vi "Extract Court (SubVI).vi"(2 "error in (no error)":errorcluster, 3 "AVI Path":path) -> (0 "error out":errorcluster, 1 "Court pixels out":u8[][](array[numeric]))   [LabVIEW 2014]
uses:
  <vilib>/vision/NI_Vision_Development_Module.lvlib
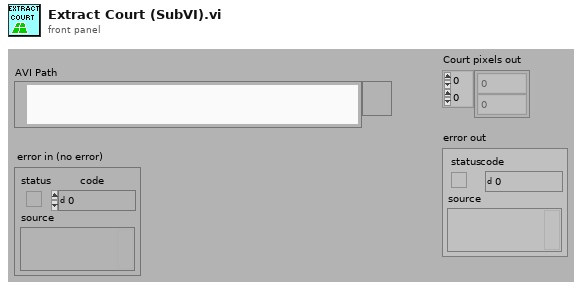
[diagram p1: front panel]
types:
  T1 = enum32{"AutoM", "Close", "Dilate", "Erode", "Gradient", "Gradient in", "Gradient out", "HitMiss", "Open", "PClose", "POpen", "Thick", "Thin"}
  T2 = typedef "Image Type" = u32
  T3 = typedef "AviRefnum.ctl" = refnum<k1>
  T4 = typedef "IMAQ Image.ctl" = refnum<image>
  T5 = cluster{"Starting Value":sgl, "Incremental Value":sgl, "Histogram":u32[]}
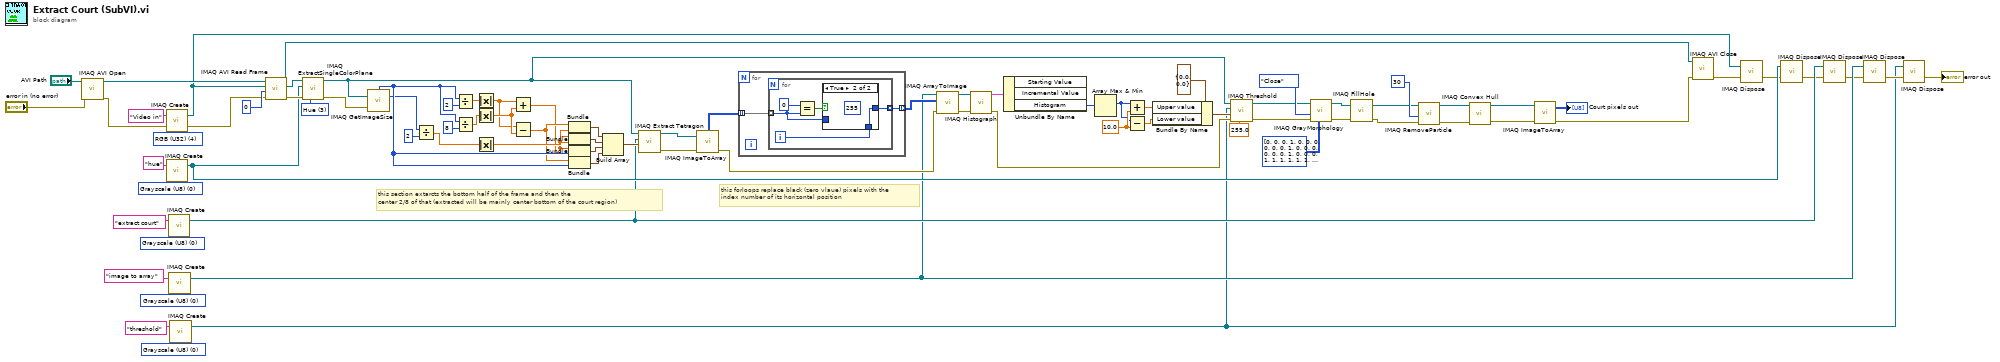
[diagram p0: block diagram]
diagram:
  w37 = 3 items=["Red", "Green", "Blue", "Hue", "Saturation", "Luminance", "Value", "Intensity"] ("Color Plane")
  w63 = sgl 10.0 ("Upper value")
  w31 = T2 0 items=["Grayscale (U8)", "Grayscale (I16)", "Grayscale (SGL)", "Complex (CSG)", "RGB (U32)", "HSL (U32)", "RGB (U64)", "Grayscale (U16)"] ("Image Type")
  w33 = T2 0 items=["Grayscale (U8)", "Grayscale (I16)", "Grayscale (SGL)", "Complex (CSG)", "RGB (U32)", "HSL (U32)", "RGB (U64)", "Grayscale (U16)"] ("Image Type")
  w29 = T2 0 items=["Grayscale (U8)", "Grayscale (I16)", "Grayscale (SGL)", "Complex (CSG)", "RGB (U32)", "HSL (U32)", "RGB (U64)", "Grayscale (U16)"] ("Image Type")
  w28 = T2 0 items=["Grayscale (U8)", "Grayscale (I16)", "Grayscale (SGL)", "Complex (CSG)", "RGB (U32)", "HSL (U32)", "RGB (U64)", "Grayscale (U16)"] ("Image Type")
  w26 = T2 4 items=["Grayscale (U8)", "Grayscale (I16)", "Grayscale (SGL)", "Complex (CSG)", "RGB (U32)", "HSL (U32)", "RGB (U64)", "Grayscale (U16)"] ("Image Type")
  # "this forloops replace black (zero vlaue) pixels with the \nindex number of its horizontal position"
  # "this section extarcts the bottom half of the frame and then the \ncenter 2/8 of that (extracted will be mainly center bottom of the court region)"
  n1 = call "IMAQ AVI Open"("error in (no error)"="error in (no error)", "AVI Path"="AVI Path") -> ("error out"=w36:errorcluster, "Avi Refnum"=w35:T3)  [unwired: 8 in]
  n2 = call "IMAQ Create"("Image Name"="Video in", "Image Type"=w26, "error in (no error)"=w36) -> ("New Image"=w21:T4, "error out"=w25:errorcluster)  [unwired: 2 in]
  n3 = call "IMAQ Create"("Image Name"="hue", "Image Type"=w28) -> ("New Image"=w20:T4)  [unwired: 3 in, 1 out]
  n4 = call "IMAQ Create"("Image Name"="extract court", "Image Type"=w33) -> ("New Image"=w19:T4)  [unwired: 3 in, 1 out]
  n5 = call "IMAQ Create"("Image Name"="image to array", "Image Type"=w31) -> ("New Image"=w18:T4)  [unwired: 3 in, 1 out]
  n6 = call "IMAQ Create"("Image Name"="threshold", "Image Type"=w29) -> ("New Image"=w2:T4)  [unwired: 3 in, 1 out]
  n7 = call "IMAQ AVI Read Frame"("error in (no error)"=w25, "Frame Number"=u32 0, "Image"=w21, "Avi Refnum"=w35) -> ("error out"=w68:errorcluster, "Image Out"=w77:T4, "Avi Refnum (duplicate)"=w22:T3)  [unwired: 4 in, 1 out]
  n8 = call "IMAQ ExtractSingleColorPlane"("Color Plane"=w37, "error in (no error)"=w68, "Image Dst"=w20, "Image Src"=w77) -> ("error out"=w69:errorcluster, "Image Dst Out"=w5:T4)  [unwired: 6 in]
  n9 = call "IMAQ GetImageSize"("Image"=w5, "error in (no error)"=w69) -> ("Y Resolution"=w39:i32, "X Resolution"=w55:i32)  [unwired: 2 in, 1 out]
  n10 = Divide(x=w39, y=2) -> (x/y=w44:dbl)
  n11 = Divide(x=w55, y=2) -> (x/y=w47:dbl)
  n12 = Divide(x=w55, y=8) -> (x/y=w46:dbl)
  n13 = Absolute Value(x=w47) -> (abs(x)=w48:dbl)
  n14 = Absolute Value(x=w46) -> (abs(x)=w49:dbl)
  n15 = Absolute Value(x=w44) -> (abs(x)=w45:dbl)
  n16 = Add(x=w48, y=w49) -> (x+y=w42:dbl)
  n17 = Subtract(x=w48, y=w49) -> (x-y=w43:dbl)
  n18 = Bundle(w43, w45) -> (w50:cluster{dbl, dbl})  [unwired: 1 in]
  n19 = Bundle(w42, w45) -> (w51:cluster{dbl, dbl})  [unwired: 1 in]
  n20 = Bundle(w42, "X Resolution"=w55) -> (w52:cluster{dbl, "X Resolution":i32})  [unwired: 1 in]
  n21 = Bundle(w43, "X Resolution"=w55) -> (w53:cluster{dbl, "X Resolution":i32})  [unwired: 1 in]
  n22 = Build Array(w50, w51, w52, w53) -> (w54:cluster{dbl, "X Resolution":dbl}[])
  n23 = call-poly "IMAQ Extract Tetragon"("Tetragon"=w54, "Image Dst"=w19, "Image Src"=w5) -> ("error out"=w65:errorcluster, "Image Dst Out"=w6:T4)  [unwired: 7 in]
  n24 = call "IMAQ ImageToArray"("error in (no error)"=w65, "Image"=w6) -> ("error out"=w83:errorcluster, "Image Pixels (U8)"=w56:u8[][])  [unwired: 2 in, 3 out]
  n25 = for {
    tunnel: w56 -> [w85] mode=indexing
    tunnel: [w84] -> w57 mode=indexing
    n26 = for {
      tunnel: w85 -> [w87] mode=indexing
      tunnel: [w88] -> w84 mode=indexing
      i -> [w86]
      n27 = Equal?(x=u8 0, y=w87) -> (x = y?=w89:bool)
      n28 = case shown="True" w89 {
        tunnel: [w91 w92] -> w88
        tunnel: w87 -> [w91 _]
        tunnel: w86 -> [_ w92]
        frame False {
        }
        frame True {
          (unwired) u8 255 ("x")
        }
      }
    }
  }
  n29 = call "IMAQ ArrayToImage"("error in (no error)"=w83, "Image Pixels (U8)"=w57, "Image"=w18) -> ("error out"=w70:errorcluster, "Image Out"=w4:T4)  [unwired: 7 in]
  n30 = call "IMAQ Histograph"("error in (no error)"=w70, "Image"=w4) -> ("error out"=w71:errorcluster, "Histogram Graph"=w58:T5)  [unwired: 6 in, 2 out]
  n31 = Unbundle By Name(w58) -> ("Histogram"=w59:u32[])  [unwired: 2 out]
  n32 = Array Max & Min(array=w59) -> (max index (indices)=w60:i32)  [unwired: 3 out]
  n33 = Add(x=w60, y=w63) -> (x+y=w66:sgl)
  n34 = Subtract(x=w60, y=w63) -> (x-y=w67:sgl)
  n35 = Bundle By Name(cluster=cluster{"Lower value":sgl, "Upper value":sgl} {"Lower value"=0.0, "Upper value"=0.0} ("Range"), "Upper value"=w66, "Lower value"=w67) -> (w61:cluster{"Lower value":sgl, "Upper value":sgl})
  n36 = call "IMAQ Threshold"("Replace Value"=sgl 255.0, "error in (no error)"=w71, "Range"=w61, "Image Dst"=w2, "Image Src"=w5) -> ("error out"=w78:errorcluster, "Image Dst Out"=w3:T4)  [unwired: 5 in]
  n37 = call "IMAQ GrayMorphology"("Structuring Element"=i32[][] [[0, 0, 0, 1, 0, 0, 0], [0, 0, 0, 1, 0, 0, 0], [0, 0, 0, 1, 0, 0, 0], [1, 1, 1, 1, 1, 1, 1], [0, 0, 0, 1, 0, 0, 0], [0, 0, 0, 1, 0, 0, 0], [0, 0, 0, 1, 0, 0, 0]], "error in (no error)"=w78, "Operation"=T1."Close", "Image Src"=w3) -> ("error out"=w75:errorcluster, "Image Dst Out"=w74:T4)  [unwired: 6 in]
  n38 = call "IMAQ FillHole"("error in (no error)"=w75, "Image Src"=w74) -> ("error out"=w79:errorcluster, "Image Dst Out"=w8:T4)  [unwired: 4 in]
  n39 = call "IMAQ RemoveParticle"("error in (no error)"=w79, "Number of Erosion"=30, "Image Src"=w8) -> ("error out"=w80:errorcluster, "Image Dst Out"=w7:T4)  [unwired: 7 in]
  n40 = call "IMAQ Convex Hull"("error in (no error)"=w80, "Image Src"=w7) -> ("error out"=w12:errorcluster, "Image Dst Out"=w1:T4)  [unwired: 8 in]
  n41 = call "IMAQ ImageToArray"("error in (no error)"=w12, "Image"=w1) -> ("error out"=w11:errorcluster, "Image Pixels (U8)"=→"Court pixels out":u8[][])  [unwired: 2 in, 3 out]
  n42 = call "IMAQ AVI Close"("error in (no error)"=w11, "Avi Refnum"=w22) -> ("error out"=w17:errorcluster)  [unwired: 9 in]
  n43 = call "IMAQ Dispose"("Image"=w21, "error in (no error)"=w17) -> ("error out"=w16:errorcluster)  [unwired: 4 in]
  n44 = call "IMAQ Dispose"("Image"=w20, "error in (no error)"=w16) -> ("error out"=w15:errorcluster)  [unwired: 4 in]
  n45 = call "IMAQ Dispose"("Image"=w19, "error in (no error)"=w15) -> ("error out"=w14:errorcluster)  [unwired: 4 in]
  n46 = call "IMAQ Dispose"("Image"=w18, "error in (no error)"=w14) -> ("error out"=w10:errorcluster)  [unwired: 4 in]
  n47 = call "IMAQ Dispose"("Image"=w2, "error in (no error)"=w10) -> ("error out"=→"error out":errorcluster)  [unwired: 4 in]
